vi "Matrix Parsing (SubVI).vi"(11 "Data Matrix In":dbl[][](array[numeric])) -> (0 "Auto Sequences":dbl[](array[numeric]), 1 "Timer":dbl[](array[numeric]), 2 "GO States":dbl[](array[numeric]), 3 "Valve States":dbl[](array[numeric]), 4 "Phase":dbl[](array[numeric]), 5 "Abort State":dbl[](array[numeric]), 6 "Blank":dbl[](array[numeric]), 8 "Bedrock":dbl[](array[numeric]), 10 "Blank 2":dbl[](array[numeric]), 12 "Blank 3":dbl[](array[numeric]), 14 "Loops":dbl[](array[numeric]), 15 "System Signals":dbl[](array[numeric]), 16 "PT Array":dbl[](array[numeric]), 17 "TC Array":dbl[](array[numeric]), 18 "LC Array":dbl[](array[numeric]), 19 "LS Array":dbl[](array[numeric]))   [LabVIEW 2020]
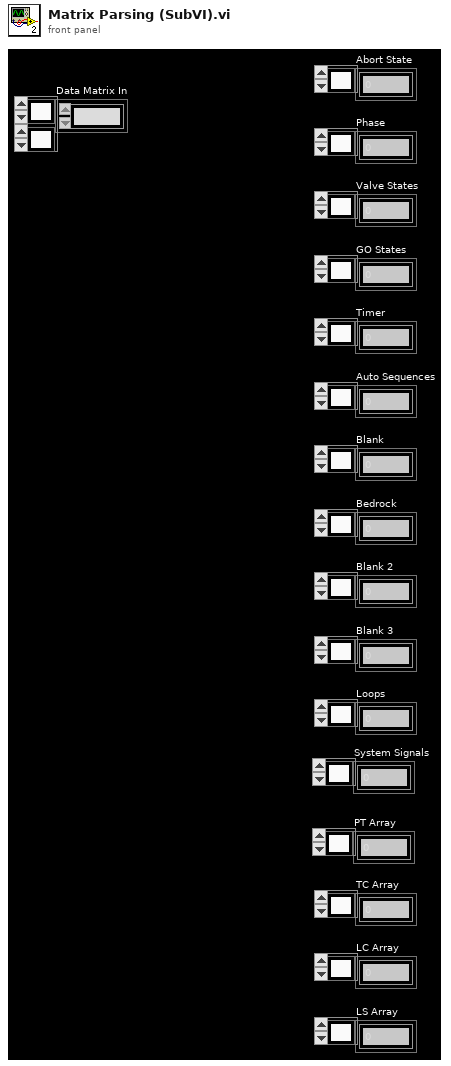
[diagram p1: front panel]
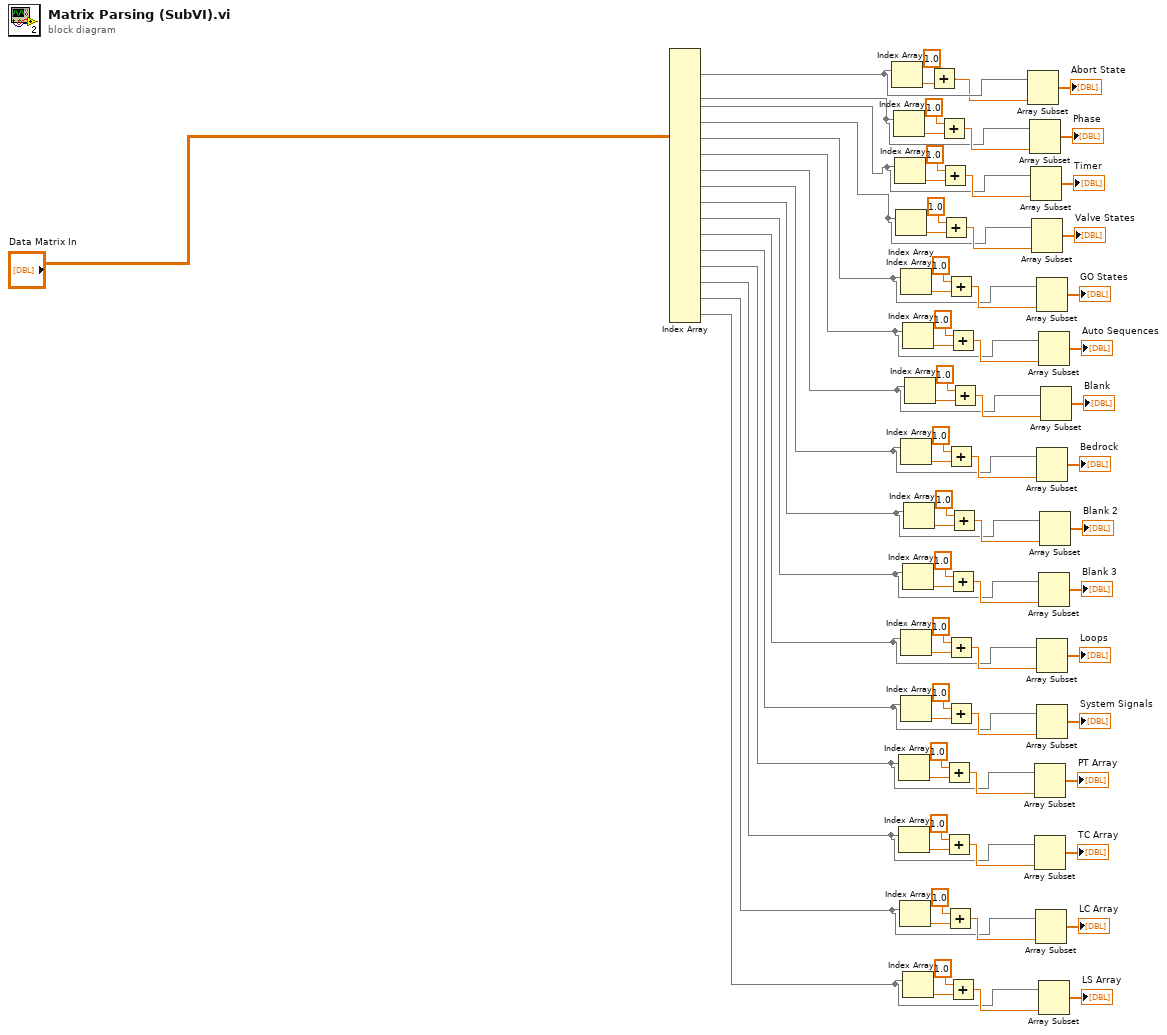
[diagram p0: block diagram]
diagram:
  n1 = Index Array(array="Data Matrix In") -> (element #1=w80:dbl[], element #2=w74:dbl[], element #3=w69:dbl[], element #4=w64:dbl[], element #5=w59:dbl[], element #6=w54:dbl[], element #7=w49:dbl[], element #8=w44:dbl[], element #9=w11:dbl[], element #10=w10:dbl[], element #11=w9:dbl[], element #12=w8:dbl[], element #13=w7:dbl[], element #14=w6:dbl[], element #15=w5:dbl[], element #16=w4:dbl[])  [unwired: 32 in]
  n2 = Index Array(array=w80) -> (element=w2:dbl)  [unwired: 1 in]
  n3 = Index Array(array=w74) -> (element=w77:dbl)  [unwired: 1 in]
  n4 = Index Array(array=w69) -> (element=w72:dbl)  [unwired: 1 in]
  n5 = Index Array(array=w64) -> (element=w67:dbl)  [unwired: 1 in]
  n6 = Index Array(array=w7) -> (element=w26:dbl)  [unwired: 1 in]
  n7 = Index Array(array=w6) -> (element=w22:dbl)  [unwired: 1 in]
  n8 = Index Array(array=w5) -> (element=w18:dbl)  [unwired: 1 in]
  n9 = Index Array(array=w59) -> (element=w62:dbl)  [unwired: 1 in]
  n10 = Index Array(array=w44) -> (element=w47:dbl)  [unwired: 1 in]
  n11 = Index Array(array=w9) -> (element=w34:dbl)  [unwired: 1 in]
  n12 = Index Array(array=w8) -> (element=w30:dbl)  [unwired: 1 in]
  n13 = Index Array(array=w54) -> (element=w57:dbl)  [unwired: 1 in]
  n14 = Index Array(array=w10) -> (element=w38:dbl)  [unwired: 1 in]
  n15 = Index Array(array=w4) -> (element=w14:dbl)  [unwired: 1 in]
  n16 = Index Array(array=w11) -> (element=w42:dbl)  [unwired: 1 in]
  n17 = Index Array(array=w49) -> (element=w52:dbl)  [unwired: 1 in]
  n18 = Add(x=1.0, y=w2) -> (x+y=w3:dbl)
  n19 = Add(x=1.0, y=w77) -> (x+y=w76:dbl)
  n20 = Add(x=1.0, y=w72) -> (x+y=w71:dbl)
  n21 = Add(x=1.0, y=w67) -> (x+y=w66:dbl)
  n22 = Add(x=1.0, y=w26) -> (x+y=w25:dbl)
  n23 = Add(x=1.0, y=w22) -> (x+y=w21:dbl)
  n24 = Add(x=1.0, y=w18) -> (x+y=w17:dbl)
  n25 = Add(x=1.0, y=w62) -> (x+y=w61:dbl)
  n26 = Add(x=1.0, y=w47) -> (x+y=w46:dbl)
  n27 = Add(x=1.0, y=w34) -> (x+y=w33:dbl)
  n28 = Add(x=1.0, y=w30) -> (x+y=w29:dbl)
  n29 = Add(x=1.0, y=w57) -> (x+y=w56:dbl)
  n30 = Add(x=1.0, y=w38) -> (x+y=w37:dbl)
  n31 = Add(x=1.0, y=w14) -> (x+y=w13:dbl)
  n32 = Add(x=1.0, y=w42) -> (x+y=w41:dbl)
  n33 = Add(x=1.0, y=w52) -> (x+y=w51:dbl)
  n34 = Array Subset(array=w80, length=w3) -> (→"Abort State":dbl[])  [unwired: 1 in]
  n35 = Array Subset(array=w74, length=w76) -> (→"Phase":dbl[])  [unwired: 1 in]
  n36 = Array Subset(array=w69, length=w71) -> (→"Timer":dbl[])  [unwired: 1 in]
  n37 = Array Subset(array=w64, length=w66) -> (→"Valve States":dbl[])  [unwired: 1 in]
  n38 = Array Subset(array=w7, length=w25) -> (→"PT Array":dbl[])  [unwired: 1 in]
  n39 = Array Subset(array=w6, length=w21) -> (→"TC Array":dbl[])  [unwired: 1 in]
  n40 = Array Subset(array=w5, length=w17) -> (→"LC Array":dbl[])  [unwired: 1 in]
  n41 = Array Subset(array=w59, length=w61) -> (→"GO States":dbl[])  [unwired: 1 in]
  n42 = Array Subset(array=w44, length=w46) -> (→"Bedrock":dbl[])  [unwired: 1 in]
  n43 = Array Subset(array=w9, length=w33) -> (→"Loops":dbl[])  [unwired: 1 in]
  n44 = Array Subset(array=w8, length=w29) -> (→"System Signals":dbl[])  [unwired: 1 in]
  n45 = Array Subset(array=w54, length=w56) -> (→"Auto Sequences":dbl[])  [unwired: 1 in]
  n46 = Array Subset(array=w10, length=w37) -> (→"Blank 3":dbl[])  [unwired: 1 in]
  n47 = Array Subset(array=w4, length=w13) -> (→"LS Array":dbl[])  [unwired: 1 in]
  n48 = Array Subset(array=w11, length=w41) -> (→"Blank 2":dbl[])  [unwired: 1 in]
  n49 = Array Subset(array=w49, length=w51) -> (→"Blank":dbl[])  [unwired: 1 in]
